vi "Move Main VI Controls.vi"(8 "error in":errorcluster, 11 "VIRef in":refnum<vi>) -> (0 "error out":errorcluster)   [LabVIEW 2018]
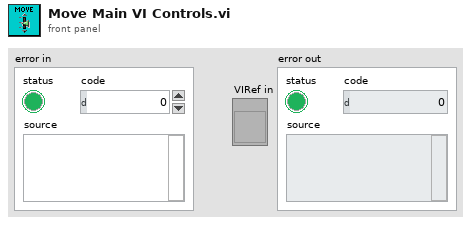
[diagram p1: front panel]
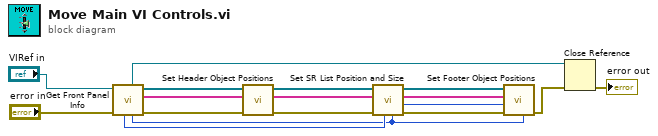
[diagram p0: block diagram]
diagram:
  n1 = call "Get Front Panel Info.vi"("error in"="error in", "VI in"="VIRef in") -> ("error out"=w17:errorcluster, "label array out"=w9:string[], "Controls[]"=w10:refnum<vi>[], "width"=w1:i16, "panel ref out"=w13:refnum<vi>, "height"=w7:i16)  [unwired: 4 in]
  n2 = call "Set Header Object Positions.vi"("error in"=w17, "label array in"=w9, "controls[] in"=w10) -> ("error out"=w8:errorcluster, "label array out"=w11:string[], "controls[] out"=w12:refnum<vi>[])  [unwired: 6 in]
  n3 = call "Set SR List Position and Size.vi"("FP.width"=w1, "FP.height"=w7, "error in"=w8, "label array in"=w11, "controls[] in"=w12) -> ("error out"=w4:errorcluster, "SR List.height"=w3:u32, "label array out"=w5:string[], "controls[] out"=w6:refnum<vi>[])  [unwired: 3 in]
  n4 = call "Set Footer Object Positions.vi"("FP.width"=w1, "error in"=w4, "SR List.height"=w3, "label array in"=w5, "controls[] in"=w6) -> ("error out"=w14:errorcluster)  [unwired: 6 in]
  n5 = Close Reference(reference=w13, error in (no error)=w14) -> (error out=→"error out":errorcluster)
